vi "Close Session.vi"(8 "error in (no error)":errorcluster, 11 "Session in":refnum<class "Plugin Session.lvclass">) -> (0 "error out":errorcluster)   [LabVIEW 2021, in "InstrumentStudio Plugin SDK.lvlib" / "Plugin Session.lvclass"]
doc: "Call this VI to close out all references created for the session and unregister the plugin session with the framework. It should be called at the end of your plugin VI after the event loop is completed as the last call in the VI."
uses:
  Plugin Session.lvclass
  Plugin Session.lvclass/Plugin Session.ctl
  Plugin Events.ctl
  Event Registration Refnum.ctl
  Read Plugin Events.vi
  Read Event Refnum.vi
  InstrumentStudio Plugin SDK.lvlib
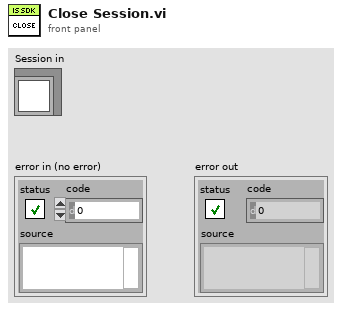
[diagram p1: front panel]
types:
  T1 = typedef "InstrumentStudio Plugin SDK.lvlib/Plugin Events.ctl" = cluster{"Shutdown":refnum<user-event>, "Project Saved":refnum<user-event>, "Stop All Outputs":refnum<user-event>, "Generic Message":refnum<user-event>, "Active Pin Map Changed":refnum<user-event>, "Selected Sites Changed":refnum<user-event>}
  T2 = typedef "InstrumentStudio Plugin SDK.lvlib/Event Registration Refnum.ctl" = refnum<event-registration>
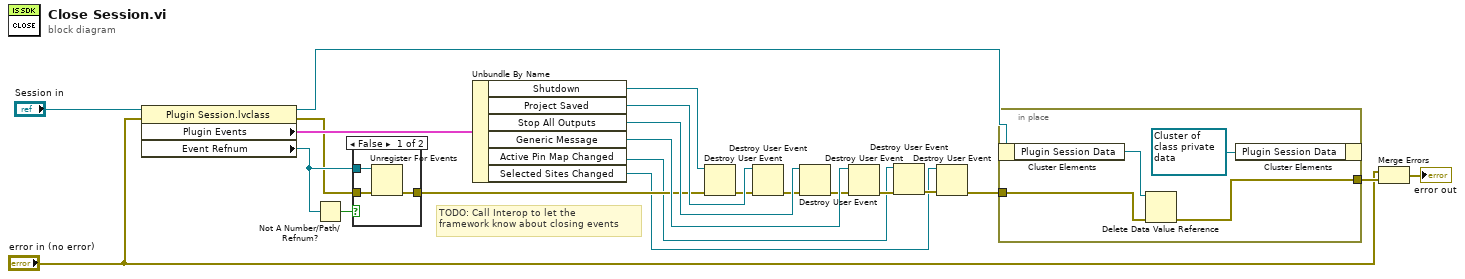
[diagram p0: block diagram]
diagram:
  # "TODO: Call Interop to let the\nframework know about closing events"
  n1 = property class="Plugin Session.lvclass"(reference="Session in", error in="error in (no error)") -> (reference out=w11:refnum<class "Plugin Session.lvclass">, error out=w10:errorcluster, "Plugin Events"=w18:T1, "Event Refnum"=w15:T2)
  n2 = Not A Number/Path/Refnum?(number/path/refnum=w15) -> (NaN/Path/Refnum?=w19:bool)
  n3 = case shown="False" w19 {
    tunnel: [w25 w26] -> w14
    tunnel: w15 -> [w24 _]
    tunnel: w10 -> [w23 w26]
    frame False {
      n4 = Unregister For Events(event registration refnum=w24, error in=w23) -> (error out=w25:errorcluster)
    }
    frame True {
    }
  }
  n5 = Unbundle By Name(w18) -> ("Shutdown"=w17:refnum<user-event>, "Project Saved"=w16:refnum<user-event>, "Stop All Outputs"=w21:refnum<user-event>, "Generic Message"=w22:refnum<user-event>, "Active Pin Map Changed"=w5:refnum<user-event>, "Selected Sites Changed"=w1:refnum<user-event>)
  n6 = Destroy User Event(user event=w17, error in=w14) -> (error out=w7:errorcluster)
  n7 = Destroy User Event(user event=w16, error in=w7) -> (error out=w9:errorcluster)
  n8 = Destroy User Event(user event=w21, error in=w9) -> (error out=w8:errorcluster)
  n9 = Destroy User Event(user event=w22, error in=w8) -> (error out=w6:errorcluster)
  n10 = Destroy User Event(user event=w5, error in=w6) -> (error out=w3:errorcluster)
  n11 = Destroy User Event(user event=w1, error in=w3) -> (error out=w2:errorcluster)
  n12 = in-place {
    in-place-border: w2 -> [w30]
    in-place-border: [w28] -> w12
    n13 = in-place-cluster #1(w11) -> ("Plugin Session Data"=w29:refnum<data-value>)
    n14 = Delete Data Value Reference(data value reference=w29, error in=w30) -> (error out=w28:errorcluster)  [unwired: 1 out]
    n15 = in-place-cluster #1("Plugin Session Data"=refnum<data-value> refnum) -> ()  [unwired: 1 out]
  }
  n16 = Merge Errors("error in (no error)", w12) -> (→"error out":errorcluster)
